vi "fpga_status.vi"(8 "error in (no error)":errorcluster, 11 "5785_2_X_400MHz_Rx_as_scop in":refnum<class "5785_2_X_400MHz_Rx_as_scop.lvclass">) -> (0 "error out":errorcluster, 2 "pulse TX status":T2, 3 "5785_2_X_400MHz_Rx_as_scop out":refnum<class "5785_2_X_400MHz_Rx_as_scop.lvclass">)   [LabVIEW 2021, in "5785_2_X_400MHz_Rx_as_scop.lvclass"]
uses:
  5785_2_X_400MHz_Rx_as_scop.lvclass
  5785_2_X_400MHz_Rx_as_scop.lvclass/5785_2_X_400MHz_Rx_as_scop.ctl
  <vilib>/Utility/error.llb/Error Cluster From Error Code.vi
  <vilib>/rvi/errors/niLvFpgaAdjustHostInterfaceError.vi
  <vilib>/rvi/interface/nirviReadWriteControl/nirviReadWriteControl.xnode
  NiFpgaLv.dll
  <vilib>/rvi/interface/Simulation/niFpgaSimulationCallBeginRW.vi
panel:
  out "pulse TX status 2":T1
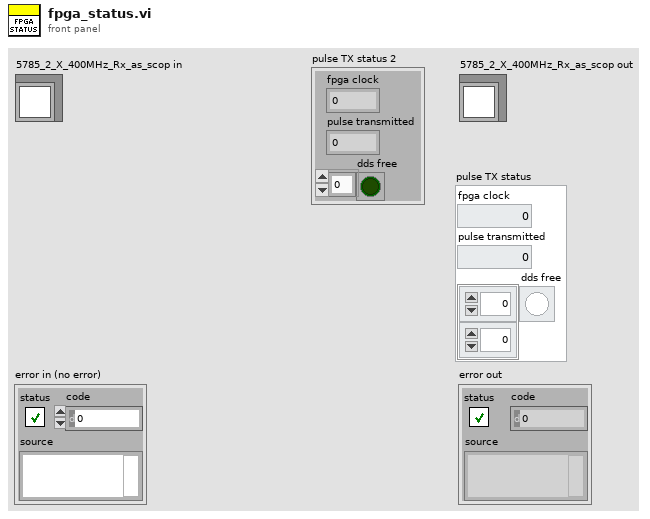
[diagram p1: front panel]
types:
  T1 = cluster{"fpga clock":u64, "pulse transmitted":u32, "dds free":bool[]}
  T2 = cluster{"fpga clock":dbl, "pulse transmitted":u32, "dds free":bool[][]}
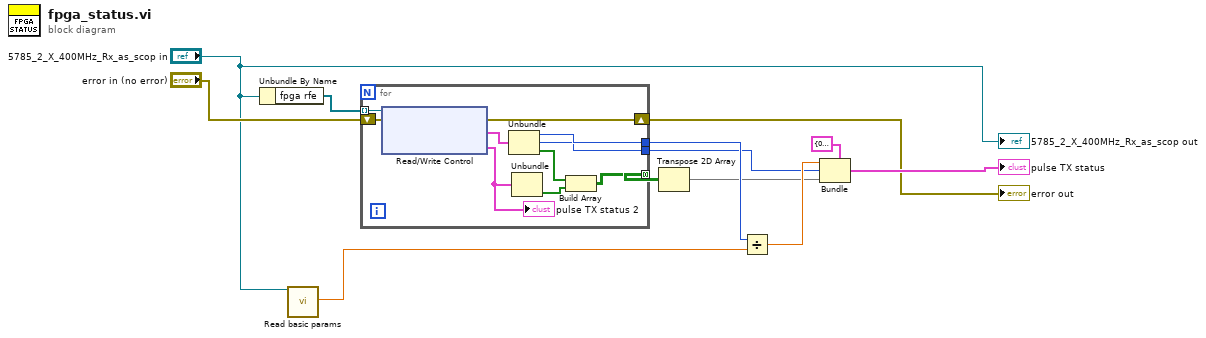
[diagram p0: block diagram]
diagram:
  n1 = Unbundle By Name("5785_2_X_400MHz_Rx_as_scop in") -> ("fpga rfe"=w12:refnum<k20>[])
  n2 = call-dynamic "Read basic params.vi"("device_type in"="5785_2_X_400MHz_Rx_as_scop in") -> ("Fs  FPGA"=w10:dbl)  [unwired: 13 in, 5 out]
  n3 = for {
    tunnel: w12 -> [w22] mode=indexing
    tunnel: [w18] -> w11
    tunnel: [w17] -> w7
    shift-right: [w20] -> w2
    shift-left: "error in (no error)" -> [w21]
    tunnel: [w15] -> w6 mode=concatenating
    n4 = xnode "Read/Write Control"("FPGA VI Reference In"=w22, "error in"=w21) -> ("error out"=w20:errorcluster, "pulse TX status"=w19:T1, "pulse TX status 2"=w14:T1)  [unwired: 1 out]
    "pulse TX status 2" <- w14
    n5 = Unbundle(w19) -> ("fpga clock"=w18:u64, "pulse transmitted"=w17:u32, "dds free"=w16:bool[])
    n6 = Unbundle(w14) -> ("dds free"=w13:bool[])  [unwired: 2 out]
    n7 = Build Array(w16, w13) -> (w15:bool[][])
  }
  "error out" <- w2
  n8 = Transpose 2D Array(2D array=w6) -> (transposed array=w5:bool[][])
  n9 = Divide(x=w11, y=w10) -> (x/y=w8:dbl)
  n10 = Bundle(cluster=T2 {"fpga clock"=0.0, "pulse transmitted"=0, "dds free"=[[FALSE, FALSE, FALSE, FALSE, FALSE, FALSE, FALSE, FALSE, FALSE, FALSE, FALSE, FALSE, FALSE, FALSE, FALSE, FALSE]]} ("pulse TX status"), "fpga clock"=w8, "pulse transmitted"=w7, "dds free"=w5) -> (→"pulse TX status":T2)
  "5785_2_X_400MHz_Rx_as_scop out" <- "5785_2_X_400MHz_Rx_as_scop in"
